vi "三列扭转文件.vi"(9 "扭转角度":dbl, 10 "扭转角度2":dbl, 11 "扭矩":dbl) -> (3 "字符串":string)   [LabVIEW 2016]
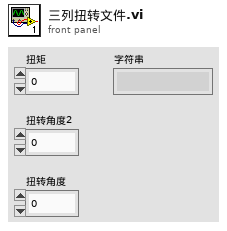
[diagram p1: front panel]
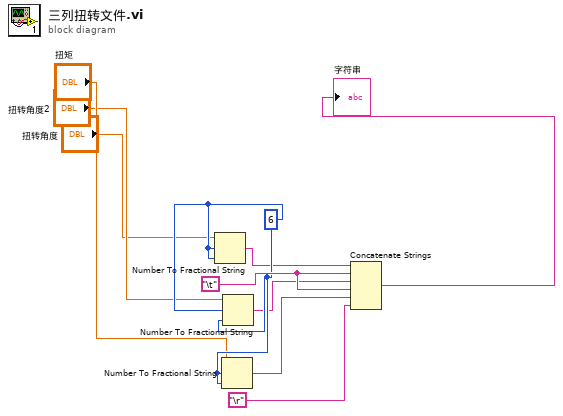
[diagram p0: block diagram]
diagram:
  w6 = i16 6 ("宽度(-)")
  w7 = "\t"
  n1 = Number To Fractional String(number="扭转角度", width (-)=w6, precision (6)=w6) -> (F-format string=w1:string)  [unwired: 1 in]
  n2 = Number To Fractional String(number="扭矩", width (-)=w6, precision (6)=w6) -> (F-format string=w8:string)  [unwired: 1 in]
  n3 = Number To Fractional String(number="扭转角度2", width (-)=w6, precision (6)=w6) -> (F-format string=w2:string)  [unwired: 1 in]
  n4 = Concatenate Strings(w1, w7, w2, w7, w8, "\r") -> (→"字符串":string)
